vi "PicoScope3000aExampleStreaming.vi"() -> ()   [LabVIEW 2016]
uses:
  ps3000aWrap.dll
  PicoScope3000aLib/PicoScope3000aAnalogChannelSettings.ctl
panel:
  out "Sample Interval (sec)":dbl format="%#.5p"
  out "AutoStopped":bool
  out "Number of Samples per Capture":i32 format="%#.6p"
  out "Total Samples":u32 format="%#.6p"
  out "TriggeredAt (Total samples)":u32 format="%#.6p"
  out "TriggeredAt (In Buffer)":u32 format="%#.6p"
  out "Triggered":bool
  out "USB 3.0 device on non-USB 3.0 Port":bool
  out "USB Powered":bool
  in  "Trigger Settings":T1={"Trigger Enabled"=FALSE, "Trigger Source"=enum."Channel A", "Trigger Threshold (volts)"=0.0, "Trigger Direction"=2, "Trigger Delay (samples)"=0, "Auto Trigger Time (ms)"=1000} {"Trigger Direction" items=["Above", "Below", "Rising", "Falling", "Rising or Falling"]}
  in  "Channel A Settings":T2={"Enabled"=TRUE, "Coupling"=1, "Range"=6, "Analogue Offset"=0.0, "Bandwidth Limit"=0} {"Bandwidth Limit" items=["Full", "20MHz"]; "Range" items=["10 mV", "20 mV", "50 mV", "100 mV", "200 mV", "500 mV", "1 V", "2 V", "5 V", "10 V", "20 V", "50 V ", "100 V"]; "Coupling" items=["AC", "DC"]}
  in  "Acquisition Settings":T3={"Auto Stop"=TRUE, "Desired Sample Interval"=1, "Pre-trigger Samples"=500000, "Post-trigger Samples"=500000, "Down-Sample Ratio"=1, "Down-Sample Mode"=0, "Overview Buffer Size"=100000, "Time Units"=3, "Four Channel Device?"=FALSE} {"Time Units" items=["Nanoseconds (ns)"=2, "Microseconds (us)"=3, "Milliseconds (ms)"=4, "Seconds (s)"=5]; "Down-Sample Mode" items=["None"=0, "Aggregate"=1, "Decimate"=2, "Average"=4]}
  in  "Apply Settings":bool
  out "Channel A":dbl[](graph)
  in  "stop":bool
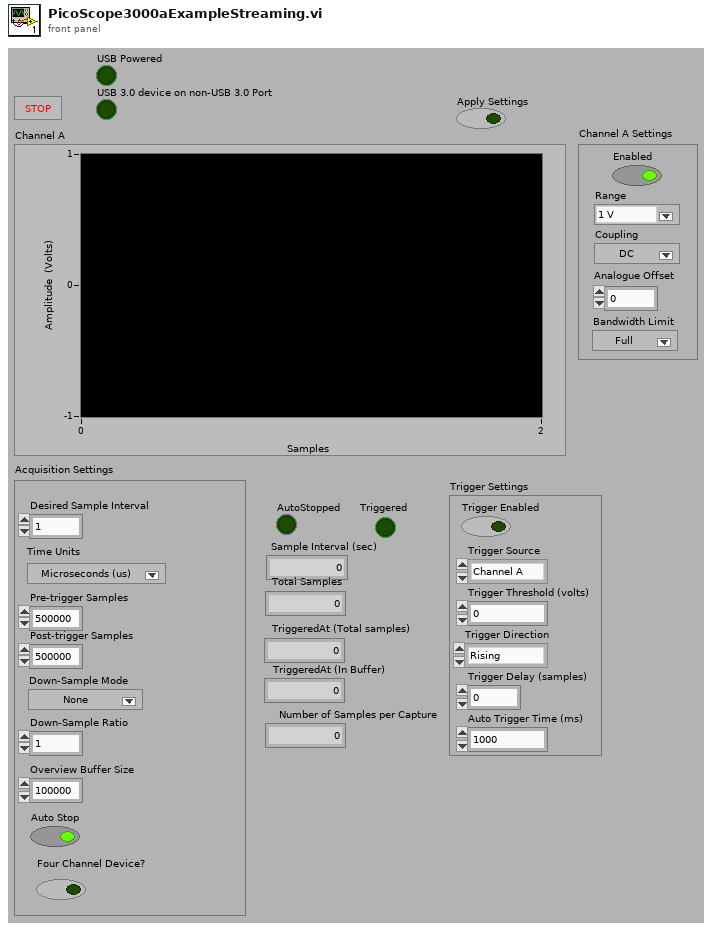
[diagram p1: front panel]
types:
  T1 = cluster{"Trigger Enabled":bool, "Trigger Source":enum32{"Channel A", "Channel B", "Channel C", "Channel D", "Ext."}, "Trigger Threshold (volts)":dbl, "Trigger Direction":u16, "Trigger Delay (samples)":u32, "Auto Trigger Time (ms)":i16}
  T2 = typedef "PicoScope3000aAnalogChannelSettings.ctl" = cluster{"Enabled":bool, "Coupling":u32, "Range":u32, "Analogue Offset":sgl, "Bandwidth Limit":u32}
  T3 = cluster{"Auto Stop":bool, "Desired Sample Interval":u32, "Pre-trigger Samples":u32, "Post-trigger Samples":u32, "Down-Sample Ratio":u32, "Down-Sample Mode":i32, "Overview Buffer Size":u32, "Time Units":u32, "Four Channel Device?":bool}
  T4 = cluster{"Driver Version":string, "USB Version":string, "Hardware":string, "Variant":string, "Batch and Serial":string, "Cal Date":string, "Kernel Version":string, "Digital HW Version":string, "Analogue HW Version":string, "MSO":bool, "Number of channels":i16}
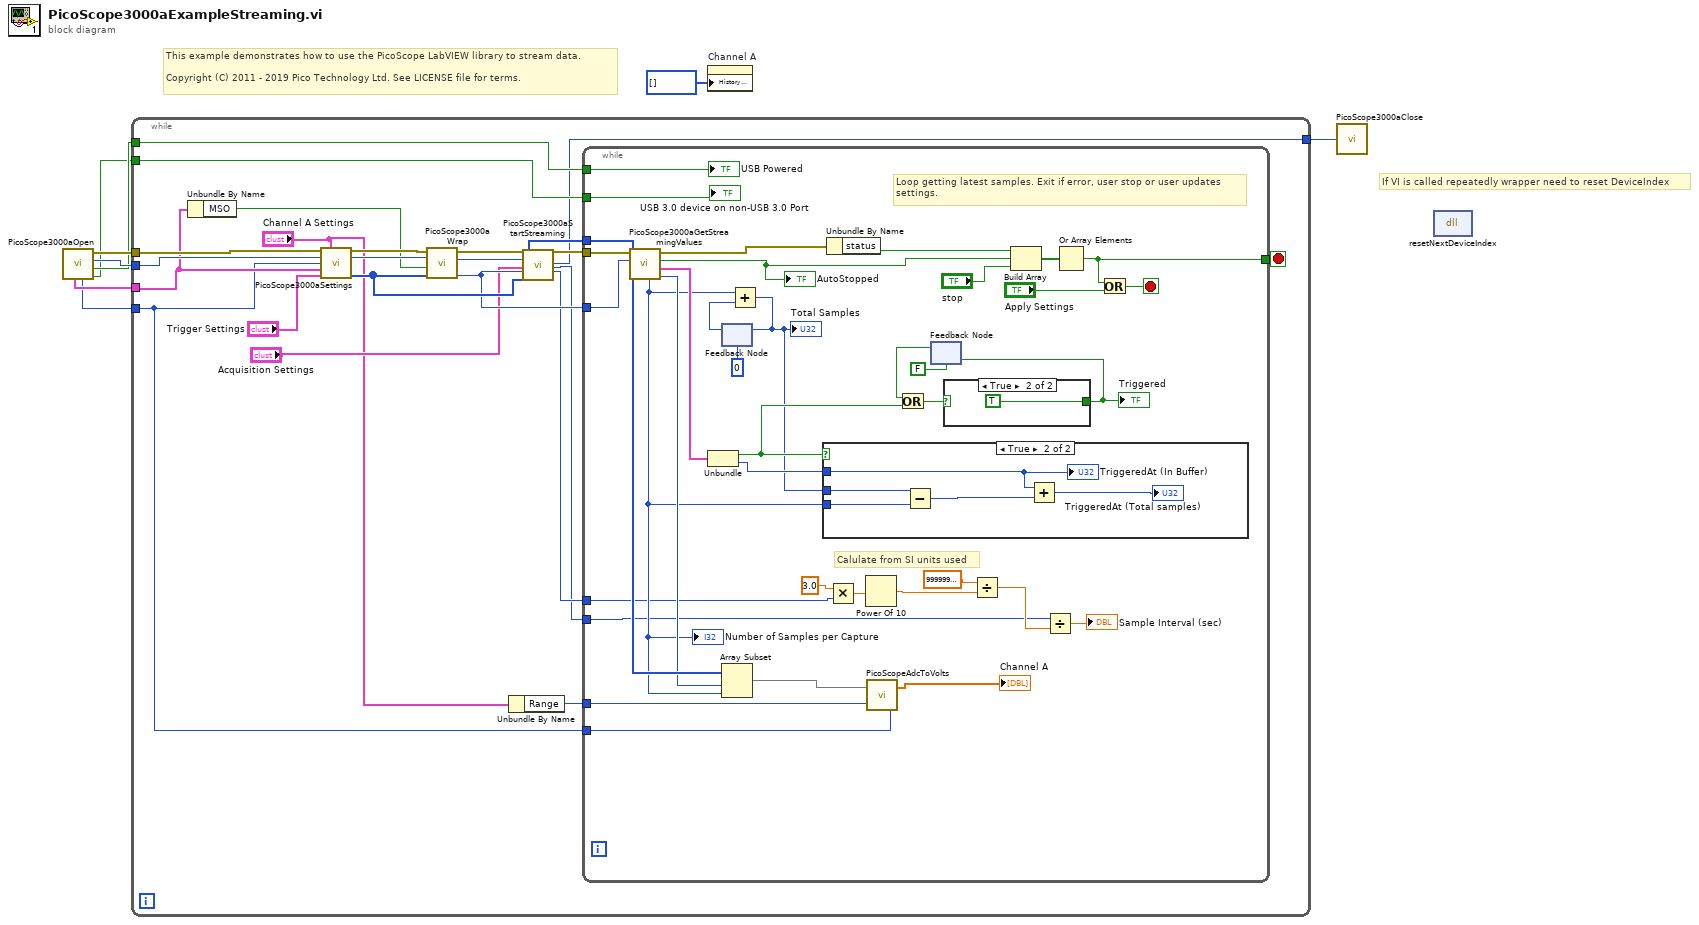
[diagram p0: block diagram]
diagram:
  # "If VI is called repeatedly wrapper need to reset DeviceIndex"
  # "This example demonstrates how to use the PicoScope LabVIEW library to stream data.\n\nCopyright (C) 2011 - 2019 Pico Technology Ltd. See LICENSE file for terms."
  n1 = call "PicoScope3000aOpen.vi"() -> ("USB 3.0 device on non-USB 3.0 Port"=w4:bool, "USB Powered"=w5:bool, "handle"=w6:i16, "error out"=w7:errorcluster, "Max ADC value"=w1:i16, "Device Info"=w2:T4)  [unwired: 6 in]
  n2 = while {
    tunnel: [w19] -> w8
    tunnel: w7 -> [w29]
    tunnel: w6 -> [w30]
    tunnel: w5 -> [w26]
    tunnel: w4 -> [w25]
    tunnel: w2 -> [w16]
    tunnel: w1 -> [w9]
    stop <- w31 stop-if-true
    n3 = Unbundle By Name(w16) -> ("MSO"=w14:bool)
    n4 = call "PicoScope3000aSettings.vi"("error in"=w29, "Channel A Settings"="Channel A Settings", "handle in"=w30, "Max_adc"=w9, "Device Info"=w16, "Trigger Settings"="Trigger Settings") -> ("error out"=w23:errorcluster, "handle out"=w21:i16, "Enabled Array"=w20:i16[])  [unwired: 7 in]
    n5 = call "PicoScope3000aWrap.vi"("Enabled Array"=w20, "MSO Device?"=w14, "handle in"=w21, "error in (no error)"=w23) -> ("deviceIndex"=w18:u16, "handle out"=w22:i16, "error out"=w24:errorcluster)  [unwired: 1 in]
    n6 = Unbundle By Name("Channel A Settings") -> ("Range"=w11:u32)
    n7 = call "PicoScope3000aStartStreaming.vi"("error in"=w24, "handle in"=w22, "Acquisition Settings"="Acquisition Settings", "deviceIndex"=w18, "Enabled Array"=w20) -> ("Channel A"=w28:i16[], "error out"=w27:errorcluster, "handle out"=w19:i16, "Sample Interval"=w12:u32, "sampleIntervalTimeUnits"=w13:i32)  [unwired: 7 in, 11 out]
    n8 = while {
      tunnel: [w57] -> w31
      tunnel: w28 -> [w66]
      tunnel: w27 -> [w63]
      tunnel: w26 -> [w56]
      tunnel: w25 -> [w55]
      tunnel: w18 -> [w62]
      tunnel: w13 -> [w40]
      tunnel: w12 -> [w36]
      tunnel: w11 -> [w34]
      tunnel: w9 -> [w33]
      stop <- w67 stop-if-true
      # "Loop getting latest samples. Exit if error, user stop or user updates \nsettings."
      # "Calulate from SI units used"
      n9 = call "PicoScope3000aGetStreamingValues.vi"("DeviceIndex"=w62, "error in"=w63) -> ("Start Index"=w64:u32, "Trigger"=w50:cluster{bool, "triggeredAt":u32}, "AutoStopped"=w59:bool, "error out"=w65:errorcluster, "Number of Samples"=w44:i32)  [unwired: 5 in]
      "Number of Samples per Capture" <- w44
      "AutoStopped" <- w59
      n10 = Unbundle(w50) -> (w49:bool, "triggeredAt"=w48:u32)
      n11 = feedback #1(u32 0) -> (w46:u32)
      n12 = Array Subset(array=w66, index=w64, length=w44) -> (w35:i16[])
      n13 = Add(x=w44, y=w46) -> (x+y=w45:u32)
      "Total Samples" <- w45
      n14 = feedback-in #1(w45) -> ()
      n15 = case shown="True" w49 {
        tunnel: w44 -> [_ w69]
        tunnel: w45 -> [_ w73]
        tunnel: w48 -> [_ w71]
        frame False {
        }
        frame True {
          n16 = Subtract(x=w73, y=w69) -> (x-y=w72:u32)
          n17 = Add(x=w71, y=w72) -> (x+y=→"TriggeredAt (Total samples)":u32)
          "TriggeredAt (In Buffer)" <- w71
        }
      }
      n18 = Unbundle By Name(w65) -> ("status"=w61:bool)
      n19 = Multiply(x=3.0, y=w40) -> (x*y=w41:dbl)
      n20 = Power Of 10(x=w41) -> (10^x=w37:dbl)
      n21 = call "PicoScopeAdcToVolts.vi"("Max_adc"=w33, "Range Index"=w34, "Data"=w35) -> ("Data"=→"Channel A":dbl[])
      n22 = feedback #2(FALSE) -> (w51:bool)
      n23 = Or(x=w51, y=w49) -> (x .or. y?=w53:bool)
      n24 = case shown="True" w53 {
        selector: w53 -> [w74 _]
        tunnel: [w74 TRUE] -> w52
        frame False {
        }
        frame True {
        }
      }
      "Triggered" <- w52
      n25 = feedback-in #2(w52) -> ()
      n26 = Divide(x=sgl 1000000000000000.0 ("y"), y=w37) -> (x/y=w39:dbl)
      n27 = Build Array(w61, w59, "stop") -> (w58:bool[])
      n28 = Divide(x=w36, y=w39) -> (x/y=→"Sample Interval (sec)":dbl)
      n29 = Or Array Elements(Boolean array=w58) -> (logical OR=w57:bool)
      n30 = Or(x=w57, y="Apply Settings") -> (x .or. y?=w67:bool)
      "USB Powered" <- w56
      "USB 3.0 device on non-USB 3.0 Port" <- w55
    }
  }
  n31 = property on="Channel A" class="WFChart (strict)"("History Data"=i16[] []) -> ()  [unwired: 2 in, 2 out]
  n32 = call "PicoScope3000aClose.vi"("handle"=w8) -> ()
  n33 = dll-call lib="ps3000aWrap.dll" fn="resetNextDeviceIndex"() -> ()  [unwired: 4 in, 2 out]
